vi "Read TracesRef.vi"(8 "error in (no error)":errorcluster, 11 "Tracer-V in":refnum<class "Tracer-V.lvclass">) -> (0 "error out":errorcluster, 2 "TracesRef":refnum<vi>, 3 "Tracer-V out":refnum<class "Tracer-V.lvclass">)   [LabVIEW 2013, in "Tracer-V.lvclass"]
uses:
  Tracer-V.lvclass
  Tracer-V.lvclass/Tracer-V.ctl
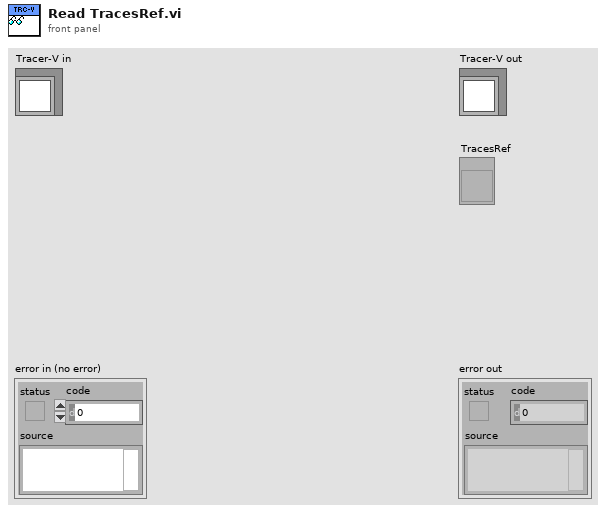
[diagram p1: front panel]
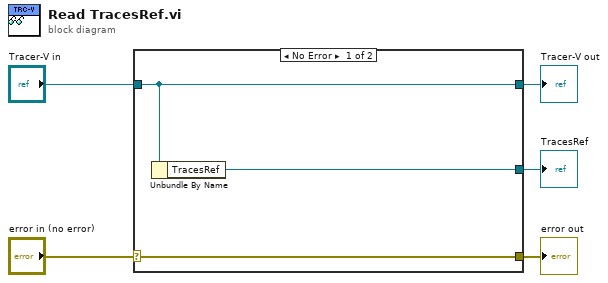
[diagram p0: block diagram]
diagram:
  n1 = case shown="No Error" "error in (no error)" {
    selector: "error in (no error)" -> [w8 w9]
    tunnel: [w8 w9] -> w4
    tunnel: [w7 w10] -> w2
    tunnel: "Tracer-V in" -> [w7 w10]
    tunnel: [w6 _] -> w1
    frame No Error {
      n2 = Unbundle By Name(w7) -> ("TracesRef"=w6:refnum<vi>)
    }
    frame Error {
    }
  }
  "error out" <- w4
  "Tracer-V out" <- w2
  "TracesRef" <- w1
